vi "remove line from table.vi"(8 "error in":errorcluster, 10 "line number":i32, 11 "operations table":T1) -> (0 "error out":errorcluster)   [LabVIEW 2013, in "CVT editor node.lvclass"]
uses:
  CVT editor node.lvclass
  table reference.ctl
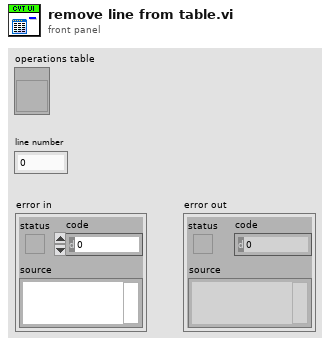
[diagram p1: front panel]
types:
  T1 = typedef "CVT editor node.lvclass/table reference.ctl" = refnum<vi>
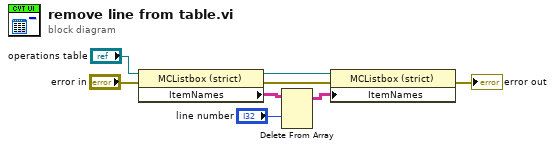
[diagram p0: block diagram]
diagram:
  n1 = property class="MCListbox (strict)"(reference="operations table", error in="error in") -> (reference out=w5:T1, error out=w4:errorcluster, "ItemNames"=w3:string[][])
  n2 = Delete From Array(array=w3, index (row)="line number") -> (array with subset deleted=w2:string[][])  [unwired: 2 in, 1 out]
  n3 = property class="MCListbox (strict)"(reference=w5, error in=w4, "ItemNames"=w2) -> (error out=→"error out":errorcluster)  [unwired: 1 out]
